vi "SetLocalWaypointDecode.vi"(11 "Payload":string) -> (2 "LocalWaypointRec":T1, 3 "string after offset":string)   [LabVIEW 2009]
uses:
  Support Files/LocalWaypointRec.ctl
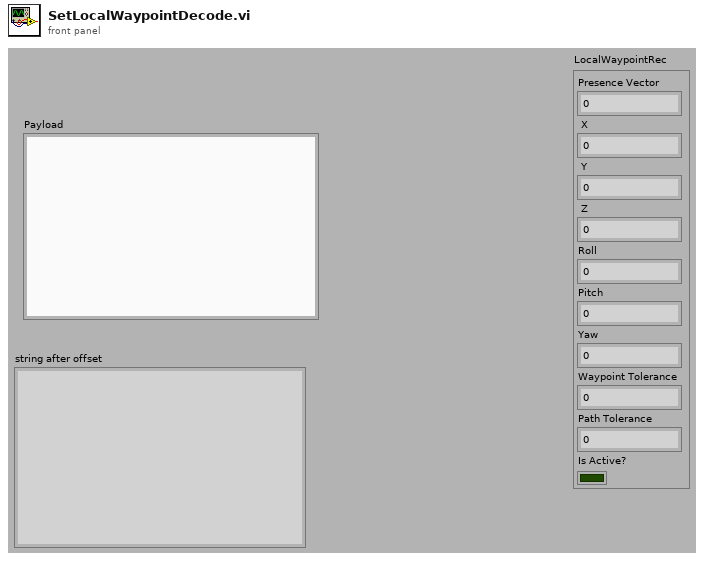
[diagram p1: front panel]
types:
  T1 = typedef "LocalWaypointRec.ctl" = cluster{"Presence Vector":u8, " X":dbl, " Y":dbl, " Z":dbl, "Roll":dbl, "Pitch":dbl, "Yaw":dbl, "Waypoint Tolerance":dbl, "Path Tolerance":dbl, "Is Active?":bool}
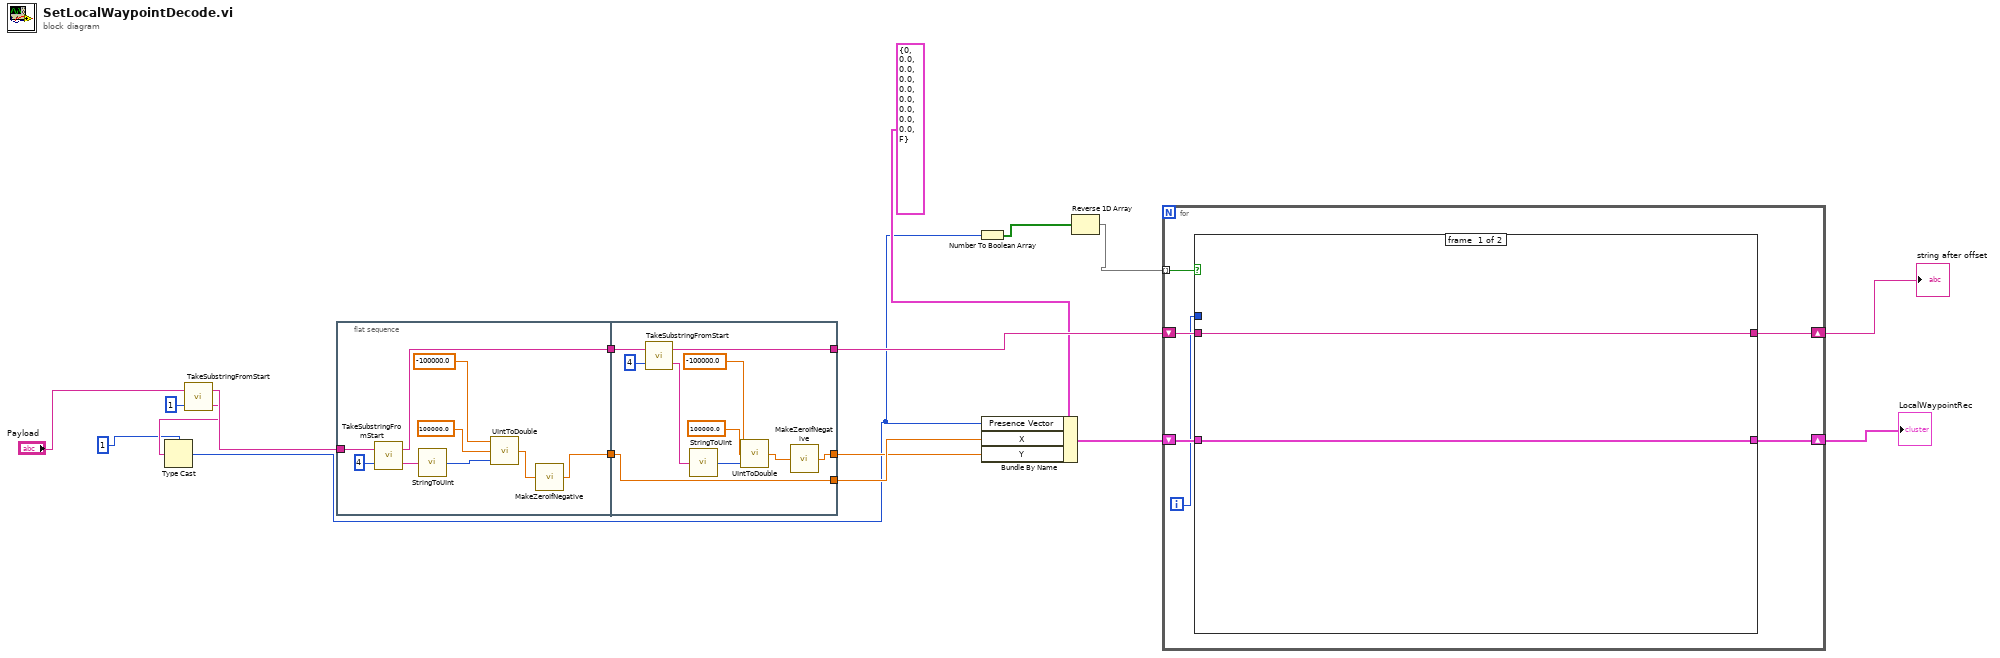
[diagram p0: block diagram]
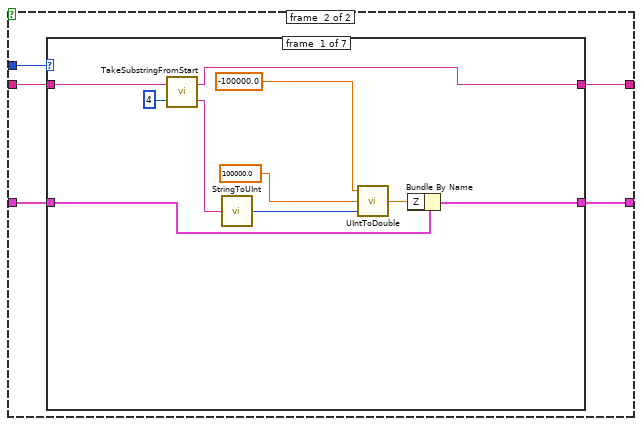
[diagram p2: hidden frame]
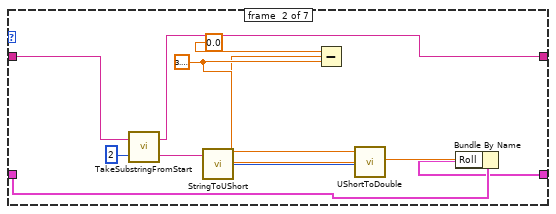
[diagram p3: hidden frame]
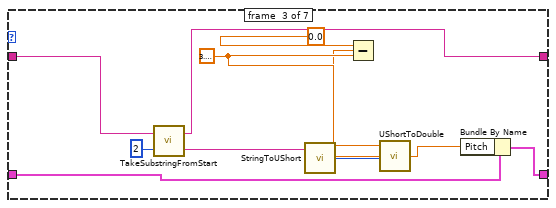
[diagram p4: hidden frame]
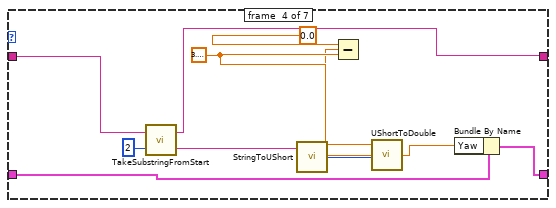
[diagram p5: hidden frame]
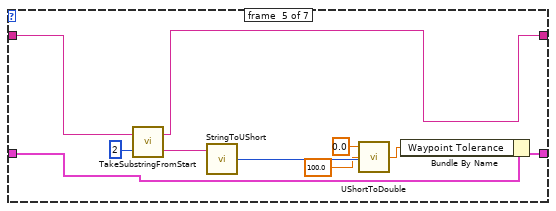
[diagram p6: hidden frame]
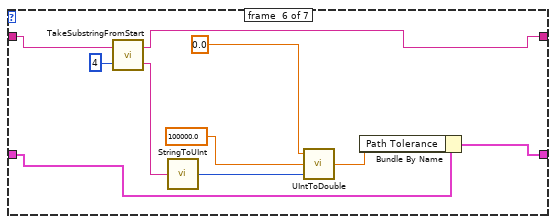
[diagram p7: hidden frame]
diagram:
  n1 = call "TakeSubstringFromStart.vi"("offset"=1, "string"="Payload") -> ("string before offset"=w5:string, "string after offset"=w6:string)
  n2 = Type Cast(type=u8 1 ("offset"), x=w5) -> (*(type *) &x=w3:u8)
  n3 = flat-sequence {
    tunnel: w6 -> [w22]
    tunnel: [w18] -> w16
    tunnel: [w20] -> w15
    tunnel: [w36] -> w17
    tunnel: w16 -> [w36]
    tunnel: w15 -> [w33]
    tunnel: [w29] -> w14
    tunnel: [w27] -> w10
    frame #0 {
      n4 = call "TakeSubstringFromStart.vi"("offset"=4, "string"=w22) -> ("string before offset"=w21:string, "string after offset"=w20:string)
      n5 = call "StringToUInt.vi"("string"=w21) -> ("UInt"=w24:u32)
      n6 = call "UIntToDouble.vi"("Value"=w24, "Max"=100000.0, "Min"=-100000.0) -> ("Number"=w19:dbl)
      n7 = call "MakeZeroIfNegative.vi"("Number"=w19) -> ("Result"=w18:dbl)
    }
    frame #1 {
      n8 = call "TakeSubstringFromStart.vi"("offset"=4, "string"=w33) -> ("string before offset"=w31:string, "string after offset"=w29:string)
      n9 = call "StringToUInt.vi"("string"=w31) -> ("UInt"=w30:u32)
      n10 = call "UIntToDouble.vi"("Value"=w30, "Max"=100000.0, "Min"=-100000.0) -> ("Number"=w28:dbl)
      n11 = call "MakeZeroIfNegative.vi"("Number"=w28) -> ("Result"=w27:dbl)
    }
  }
  n12 = Number To Boolean Array(number=w3) -> (Boolean array=w2:bool[])
  n13 = Bundle By Name(cluster=T1 {"Presence Vector"=0, " X"=0.0, " Y"=0.0, " Z"=0.0, "Roll"=0.0, "Pitch"=0.0, "Yaw"=0.0, "Waypoint Tolerance"=0.0, "Path Tolerance"=0.0, "Is Active?"=FALSE} ("LocalWaypointRec"), "Presence Vector"=w3, "X"=w17, "Y"=w10) -> (w12:T1)
  n14 = Reverse 1D Array(array=w2) -> (reversed array=w1:bool[])
  n15 = for {
    tunnel: w1 -> [w42] mode=indexing
    shift-right: [w39] -> w13
    shift-left: w12 -> [w38]
    shift-right: [w40] -> w9
    shift-left: w14 -> [w41]
    i -> [w37]
    n16 = case shown="False" w42 {
      tunnel: w41 -> [w44 w49]
      tunnel: [w44 w48] -> w40
      tunnel: [w43 w47] -> w39
      tunnel: w38 -> [w43 w46]
      tunnel: w37 -> [_ w45]
      frame #0 {
      }
      frame #1 {
        n17 = case shown="3" w45 {
          tunnel: w49 -> [w59 w70 w74 w85 w98 w106 w114]
          tunnel: [w57 w68 w75 w84 w97 w105 w114] -> w48
          tunnel: [w50 w62 w71 w82 w95 w103 w113] -> w47
          tunnel: w46 -> [w51 w63 w72 w83 w96 w104 w113]
          frame #0 {
            n18 = call "TakeSubstringFromStart.vi"("offset"=4 ("reduce by"), "string"=w59) -> ("string before offset"=w56:string, "string after offset"=w57:string)
            n19 = call "StringToUInt.vi"("string"=w56) -> ("UInt"=w55:u32)
            n20 = call "UIntToDouble.vi"("Value"=w55, "Max"=100000.0, "Min"=-100000.0) -> ("Number"=w52:dbl)
            n21 = Bundle By Name(cluster=w51, "Z"=w52) -> (w50:T1)
          }
          frame #1 {
            w67 = 3.141592653589793
            n22 = call "TakeSubstringFromStart.vi"("offset"=2, "string"=w70) -> ("string before offset"=w61:string, "string after offset"=w68:string)
            n23 = call "StringToUShort.vi"("string"=w61) -> ("UShort"=w60:u16)
            n24 = Subtract(x=0.0, y=w67) -> (x-y=w66:dbl)
            n25 = call "UShortToDouble.vi"("Value"=w60, "Max"=w67, "Min"=w66) -> ("Number"=w64:dbl)
            n26 = Bundle By Name(cluster=w63, "Roll"=w64) -> (w62:T1)
          }
          frame #2 {
            w80 = 3.141592653589793
            n27 = call "TakeSubstringFromStart.vi"("offset"=2, "string"=w74) -> ("string before offset"=w77:string, "string after offset"=w75:string)
            n28 = call "StringToUShort.vi"("string"=w77) -> ("UShort"=w76:u16)
            n29 = Subtract(x=0.0, y=w80) -> (x-y=w79:dbl)
            n30 = call "UShortToDouble.vi"("Value"=w76, "Max"=w80, "Min"=w79) -> ("Number"=w73:dbl)
            n31 = Bundle By Name(cluster=w72, "Pitch"=w73) -> (w71:T1)
          }
          frame #3 {
            w91 = 3.141592653589793
            n32 = call "TakeSubstringFromStart.vi"("offset"=2, "string"=w85) -> ("string before offset"=w88:string, "string after offset"=w84:string)
            n33 = call "StringToUShort.vi"("string"=w88) -> ("UShort"=w87:u16)
            n34 = Subtract(x=0.0, y=w91) -> (x-y=w90:dbl)
            n35 = call "UShortToDouble.vi"("Value"=w87, "Max"=w91, "Min"=w90) -> ("Number"=w86:dbl)
            n36 = Bundle By Name(cluster=w83, "Yaw"=w86) -> (w82:T1)
          }
          frame #4 {
            n37 = call "TakeSubstringFromStart.vi"("offset"=2, "string"=w98) -> ("string before offset"=w101:string, "string after offset"=w97:string)
            n38 = call "StringToUShort.vi"("string"=w101) -> ("UShort"=w100:u16)
            n39 = call "UShortToDouble.vi"("Value"=w100, "Max"=100.0, "Min"=0.0) -> ("Number"=w99:dbl)
            n40 = Bundle By Name(cluster=w96, "Waypoint Tolerance"=w99) -> (w95:T1)
          }
          frame #5 {
            n41 = call "TakeSubstringFromStart.vi"("offset"=4 ("reduce by"), "string"=w106) -> ("string before offset"=w111:string, "string after offset"=w105:string)
            n42 = call "StringToUInt.vi"("string"=w111) -> ("UInt"=w110:u32)
            n43 = call "UIntToDouble.vi"("Value"=w110, "Max"=100000.0, "Min"=0.0) -> ("Number"=w107:dbl)
            n44 = Bundle By Name(cluster=w104, "Path Tolerance"=w107) -> (w103:T1)
          }
          frame #6 {
          }
        }
      }
    }
  }
  "LocalWaypointRec" <- w13
  "string after offset" <- w9
